vi "ExitApp.vi"() -> ()   [LabVIEW 2017]
uses:
  controls/ConsumerCmd.ctl
  controls/ConsumerCtl.ctl
  controls/UpdateMessageCmd.ctl
  controls/UpdateMessageCtl.ctl
  controls/DisplayCmd.ctl
  controls/DisplayCtl.ctl
  controls/DisplayCommanda.ctl
  Downloads/ATM Simulator/Controls/DisplayControl.ctl
panel:
  in  "Display Queue in":refnum<queue>
  out "error out":errorcluster
  in  "error in (no error)":errorcluster
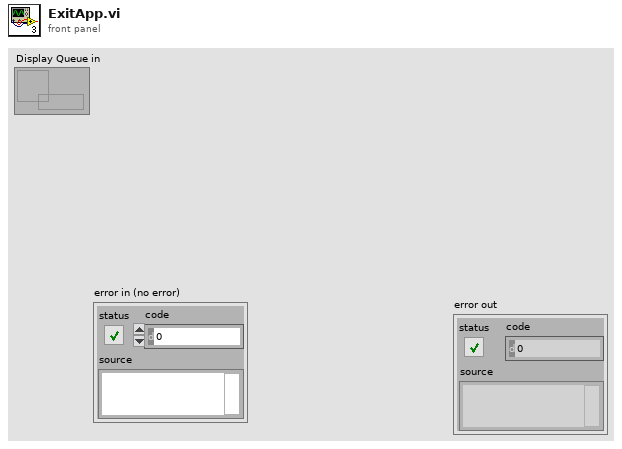
[diagram p1: front panel]
types:
  T1 = typedef "DisplayCtl.ctl" = cluster{"Command":T2, "Data":variant}
  T2 = typedef "DisplayCmd.ctl" = enum16{"Initialize", "Enable/Disable Controls", "FocusCursor", "UpdateMessage", "Update Menus", "Finish Operation", "Exit", "Clean User Input"}
  T3 = typedef "UpdateMessageCtl.ctl" = cluster{"Command":T4, "Data":variant}
  T4 = typedef "UpdateMessageCmd.ctl" = enum16{"Welcome", "Main Menu", "Account Failed", "Session Terminated", "Deposit", "Deposit Complete", "Withdrawal", "Withdrawal Complete"}
  T5 = typedef "ConsumerCtl.ctl" = cluster{"Command":T6, "Data":variant}
  T6 = typedef "ConsumerCmd.ctl" = enum16{"Initialize", "User Input", "Start operation", "Left Button", "Right Button", "Exit"}
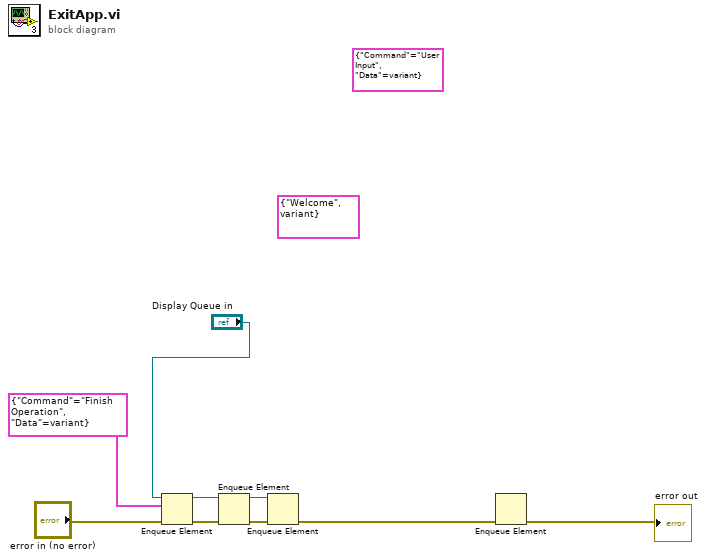
[diagram p0: block diagram]
diagram:
  (unwired) T3 {"Command"=enum."Welcome", "Data"=variant} ("Cluster")
  (unwired) T5 {"Command"=enum."User Input", "Data"=variant} ("Cluster")
  n1 = Enqueue Element(queue="Display Queue in", element=T1 {"Command"=enum."Finish Operation", "Data"=variant} ("Cluster"), error in (no error)="error in (no error)") -> (queue out=w4:refnum<queue>, error out=w8:errorcluster)  [unwired: 1 in, 1 out]
  n2 = Enqueue Element(queue=w4, error in (no error)=w8) -> (queue out=w3:refnum<queue>, error out=w9:errorcluster)  [unwired: 2 in, 1 out]
  n3 = Enqueue Element(queue=w3, error in (no error)=w9) -> (error out=w7:errorcluster)  [unwired: 2 in, 2 out]
  n4 = Enqueue Element(error in (no error)=w7) -> (error out=→"error out":errorcluster)  [unwired: 3 in, 2 out]
